vi "Common Split Bytes.vi"(11 "Double":dbl) -> (1 "Most Significant Byte":u8 format="%x", 2 "Intermediate Byte":u8 format="%x", 3 "Less Significant Byte":u8 format="%x")   [LabVIEW 2011, in "LNLS Control VIs.lvlib"]
uses:
  LNLS Control VIs.lvlib
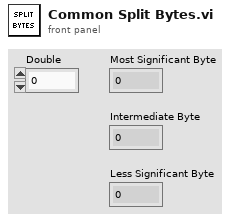
[diagram p1: front panel]
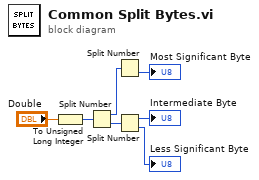
[diagram p0: block diagram]
diagram:
  n1 = To Unsigned Long Integer(number="Double") -> (unsigned 32bit integer=w2:u32)
  n2 = Split Number(x=w2) -> (hi(x)=w6:u16, lo(x)=w3:u16)
  n3 = Split Number(x=w6) -> (lo(x)=→"Most Significant Byte":u8)  [unwired: 1 out]
  n4 = Split Number(x=w3) -> (hi(x)=→"Intermediate Byte":u8, lo(x)=→"Less Significant Byte":u8)
